vi "Sine Integral.vi"(3 "x":dbl format="%.2f") -> (1 "Si(x)":dbl format="%.2f")   [LabVIEW 2024, in "NI_Gmath.lvlib"]
doc: "<p>Evaluates the sine integral for any real number <strong>x</strong>.</p>"
uses:
  NI_Gmath.lvlib
  <resource>/lvanlys.dll
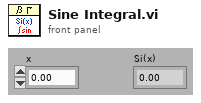
[diagram p1: front panel]
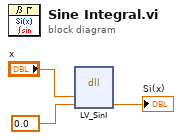
[diagram p0: block diagram]
diagram:
  n1 = dll-call lib="C:/Program Files (x86)/National Instruments/LabVIEW 2024/resource/lvanlys.*" fn="LV_SinI"("x"="x", "SinI(x)"=0.0 ("cosI")) -> ("SinI(x)"=→"Si(x)":dbl)  [unwired: 5 in, 2 out]
